vi "ReadTestType.vi"(8 "error in (no error)":errorcluster, 11 "列名":string) -> (0 "error out":errorcluster, 3 "输出 1":dbl)   [LabVIEW 2014]
uses:
  <vilib>/addons/database/Connection.llb/DB Tools Open Connec (String).vi
  <vilib>/addons/database/Connection.llb/Conn Execute.vi
  <vilib>/addons/database/Recordset.llb/Rec Fetch Recordset Data (R).vi
  <vilib>/addons/database/Recordset.llb/Rec Destroy - Connection.vi
  <vilib>/addons/database/_DB Variant To Data/Database Variant To Data.xnode
  <vilib>/addons/database/NI_Database_API.lvlib
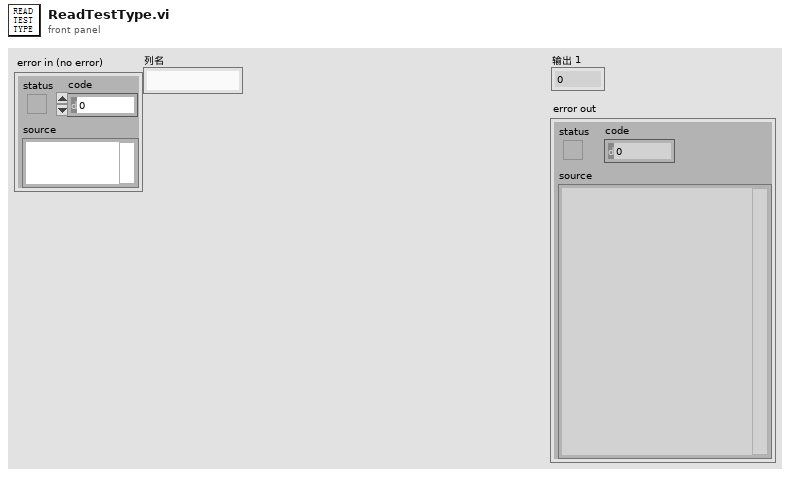
[diagram p1: front panel]
types:
  T1 = typedef "NI_Database_API.lvlib/Conn ObjectReference.ctl" = refnum<k1>
  T2 = typedef "NI_Database_API.lvlib/Rec ObjectReference.ctl" = refnum<k1>
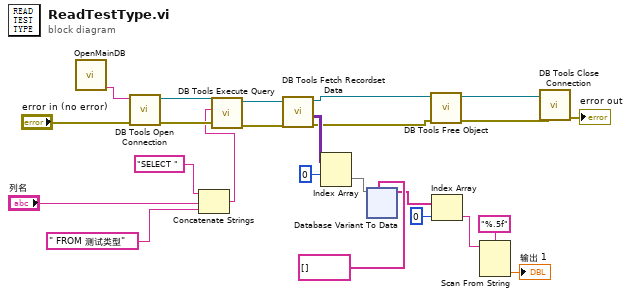
[diagram p0: block diagram]
diagram:
  n1 = call "OpenMainDB.vi"() -> ("头信息"=w24:string)  [unwired: 11 in]
  n2 = call-poly <vilib>:"DB Tools Open Connection.vi"("error in (no error)"="error in (no error)", "connection information"=w24) -> ("error out"=w21:errorcluster, "connection reference"=w22:T1)  [unwired: 6 in]
  n3 = Concatenate Strings("SELECT ", "列名", " FROM 测试类型") -> (w17:string)
  n4 = call-poly <vilib>:"DB Tools Execute Query.vi"("error in (no error)"=w21, "SQL query"=w17, "connection reference"=w22) -> ("error out"=w15:errorcluster, "recordset reference"=w16:T2)  [unwired: 5 in]
  n5 = call-poly <vilib>:"DB Tools Fetch Recordset Data.vi"("error in (no error)"=w15, "recordset reference"=w16) -> ("error out"=w4:errorcluster, "recordset data"=w14:variant[][], "recordset reference out"=w5:T2)  [unwired: 3 in]
  n6 = Index Array(array=w14, index (row)=0 ("索引 (行)")) -> (element=w12:variant[])  [unwired: 1 in]
  n7 = xnode "Database Variant To Data"("database variant"=w12, "type"=string[] []) -> ("data"=w10:string[])  [unwired: 1 in, 1 out]
  n8 = call-poly <vilib>:"DB Tools Free Object.vi"("error in (no error)"=w4, "recordset reference"=w5) -> ("error out"=w2:errorcluster, "connection reference"=w3:T1)  [unwired: 8 in]
  n9 = Index Array(array=w10, index=0 ("索引")) -> (element=w8:string)
  n10 = Scan From String(format string="%.5f" ("格式字符串"), input string=w8) -> (output 1=→"输出 1":dbl)  [unwired: 3 in, 3 out]
  n11 = call <vilib>:"DB Tools Close Connection.vi"("error in (no error)"=w2, "connection reference"=w3) -> ("error out"=→"error out":errorcluster)  [unwired: 5 in]
